vi "BASICS.vi"(4 "Offset":dbl(knob) min=0.0 max=50.0 step=0.1 scale=0.0..50.0, 5 "Frequency units":u32(ring) items=["Hz"=1, "KHz"=1000, "MHz"=1000000], 6 "Amplitude":dbl(knob) scale=0.0..10.0, 7 "Frequency":dbl(knob) min=0.0 max=1000.0 step=1.0 scale=2.0..1000.0, 8 "error in":errorcluster, 10 "Waveform":u16(ring) items=["SIN", "SQU", "TRI", "RAMP", "NOI", "DC", "USER"], 11 "Address":string) -> (0 "error out":errorcluster, 2 "Send command":string, 3 "Address (out)":string)   [LabVIEW 2024]
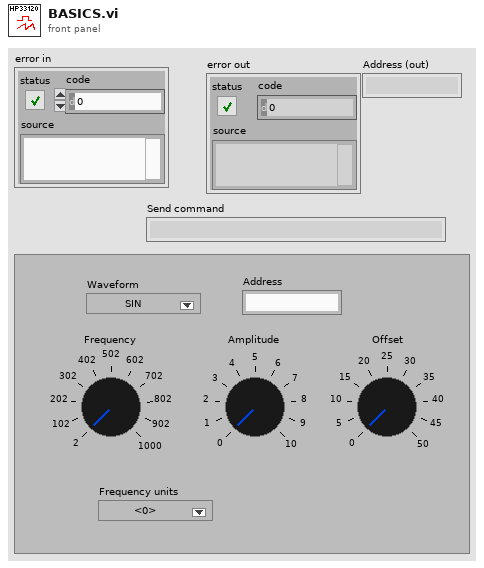
[diagram p1: front panel]
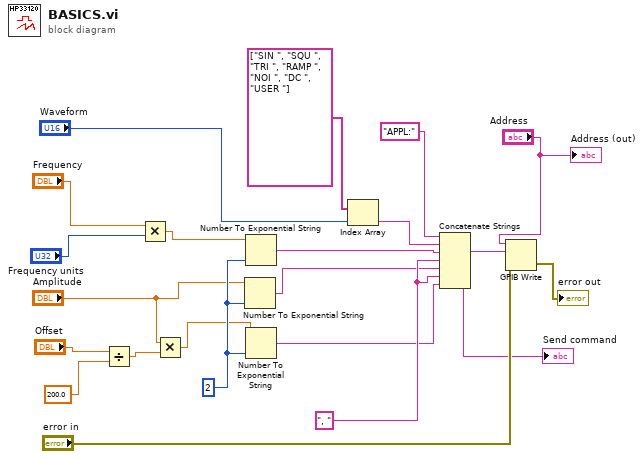
[diagram p0: block diagram]
diagram:
  w13 = ", "
  w19 = 2
  n1 = Divide(x="Offset", y=200.0) -> (x/y=w9:dbl)
  n2 = Multiply(x="Frequency", y="Frequency units") -> (x*y=w4:dbl)
  n3 = Multiply(x="Amplitude", y=w9) -> (x*y=w8:dbl)
  n4 = Number To Exponential String(number="Amplitude", precision (6)=w19) -> (E-format string=w11:string)  [unwired: 2 in]
  n5 = Number To Exponential String(number=w4, precision (6)=w19) -> (E-format string=w14:string)  [unwired: 2 in]
  n6 = Number To Exponential String(number=w8, precision (6)=w19) -> (E-format string=w12:string)  [unwired: 2 in]
  n7 = Index Array(array=string[] ["SIN ", "SQU ", "TRI ", "RAMP ", "NOI ", "DC ", "USER "], index="Waveform") -> (element=w15:string)
  n8 = Concatenate Strings("APPL:" ("Address 2"), w15, w14, w13, w11, w13, w12) -> (w17:string)
  "Send command" <- w17
  n9 = GPIB Write(0:"Address", 1:w17, 3:"error in") -> (6:→"error out":errorcluster)  [unwired: 2 in, 1 out]
  "Address (out)" <- "Address"
